vi "Orca Data Spooler Update Log Copy Status.vi"(0 "Transfer Log":path, 11 "Copy Success":bool) -> (15 "Update Error":errorcluster)   [LabVIEW 2016]
uses:
  Orca Data Spooler Type Defs/Orca Data Spooler Transfer Log Type.ctl
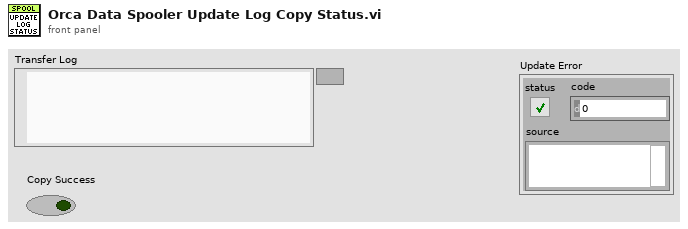
[diagram p1: front panel]
types:
  T1 = typedef "Orca Data Spooler Transfer Log Type.ctl" = cluster{"File Name":string, "Status":string}
  T2 = enum16{"open", "replace", "create", "open or create", "replace or create", "replace or create with confirmation"}
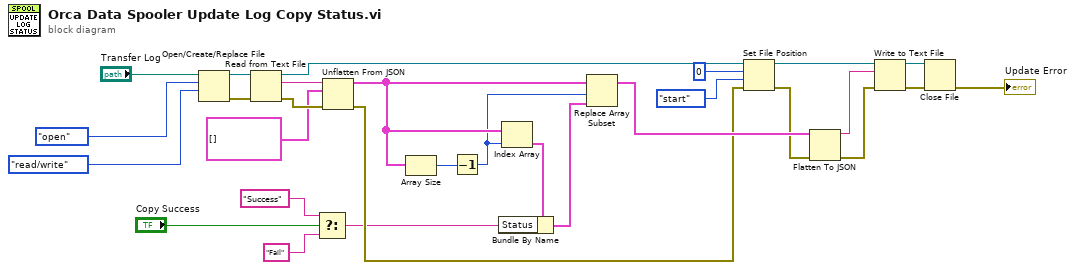
[diagram p0: block diagram]
diagram:
  n1 = Open/Create/Replace File(file path (use dialog)="Transfer Log", operation (0:open)=T2."open", access (0:read/write)=enum16{"read/write", "read-only", "write-only"}."read/write") -> (refnum out=w27:refnum<file>, error out=w26:errorcluster)  [unwired: 3 in, 1 out]
  n2 = Read from Text File(file (use dialog)=w27, error in=w26) -> (refnum out=w23:refnum<file>, text=w25:string, error out=w24:errorcluster)  [unwired: 2 in, 1 out]
  n3 = Select(t="Success", s="Copy Success", f="Fail") -> (s? t:f=w3:string)
  n4 = Unflatten From JSON(JSON string=w25, type and defaults=T1[] [], error in (no error)=w24) -> (value=w13:T1[], error out=w6:errorcluster)  [unwired: 4 in]
  n5 = Array Size(array=w13) -> (size(s)=w14:i32)
  n6 = Decrement(x=w14) -> (x-1=w12:i32)
  n7 = Index Array(array=w13, index=w12) -> (element=w11:T1)
  n8 = Bundle By Name(cluster=w11, "Status"=w3) -> (w10:T1)
  n9 = Replace Array Subset(array=w13, new element=w10, index=w12) -> (w9:T1[])
  n10 = Set File Position(offset (in bytes) (0)=i64 0, refnum=w23, from (0:start)=enum16{"start", "end", "current"}."start", error in=w6) -> (refnum out=w15:refnum<file>, error out=w7:errorcluster)
  n11 = Flatten To JSON(anything=w9, error in (no error)=w7) -> (JSON string=w21:string, 11:w18:errorcluster)  [unwired: 1 in]
  n12 = Write to Text File(file (use dialog)=w15, text=w21, error in=w18) -> (refnum out=w20:refnum<file>, error out=w19:errorcluster)  [unwired: 1 in, 1 out]
  n13 = Close File(refnum=w20, error in=w19) -> (error out=→"Update Error":errorcluster)  [unwired: 1 out]
